vi "Gui4.vi"() -> ()   [LabVIEW 2009]
uses:
  <vilib>/rvi/interface/nirviOpenFPGA/nirviOpenFPGA.xnode
  FPGA Bitfiles/Athena Brain.lvproj_FPGA Target 2_Gray's Mod Motor C~4B.lvbitx
  FPGA/Gray's Mod Motor Controler.vi
  <vilib>/userDefined/High Color/nirio_resource_hc.ctl
  <vilib>/rvi/interface/nirviReadWriteControl/nirviReadWriteControl.xnode
  NiRioSrv.dll
  <vilib>/Utility/error.llb/Error Cluster From Error Code.vi
  <vilib>/rvi/errors/niLvFpgaWhatHappensToTopLevelVI.ctl
  <vilib>/rvi/interface/common/niFpgaNodeNameForErrorReporting.ctl
  <vilib>/rvi/errors/niLvFpgaAdjustHostInterfaceError.vi
  <vilib>/rvi/interface/nirviMethod/nirviMethod.xnode
  <vilib>/rvi/interface/nirviCloseFPGA/nirviCloseFPGA.xnode
  <vilib>/FPGAPlugInAG/sbRIO-9642/nirviIntfOpen_sbRIO-9642.vi
  <vilib>/Utility/error.llb/Merge Errors.vi
  <vilib>/LabVIEW Targets/FPGA/RIO/nirio_HostInterface/nirio_Reset.vi
  <vilib>/LabVIEW Targets/FPGA/RIO/nirio_HostInterface/nirio_DMAStopAll.vi
  <vilib>/LabVIEW Targets/FPGA/RIO/nirio_HostInterface/nirio_DisableInterrupts.vi
  <vilib>/RVI Host/nirviSupport.llb/nirviErrorClusterFromErrorCode.vi
  <vilib>/FPGAPlugInAG/sbRIO-9642/nirviIntfClose_sbRIO-9642.vi
panel:
  out "Restart Loops":bool=TRUE
  in  "Reset Fpga":bool
  in  "stop":bool
  in  "Lidar Enable":bool
  in  "Lidar Output Command":fxp<+/-,20,5> format="%.17g"
  out "Lidar Output Voltage":fxp<+/-,20,5> format="%.17g"
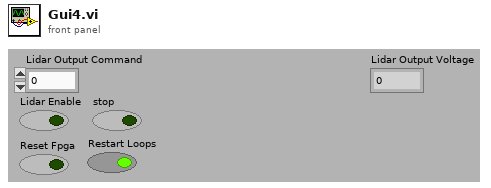
[diagram p1: front panel]
types:
  T1 = typedef "niFpgaNodeNameForErrorReporting.ctl" = enum16{"Open FPGA VI Reference", "Read/Write Control", "Invoke Method: Abort", "Invoke Method: Acknowledge IRQ", "Invoke Method: Download", "Invoke Method: FIFO.Configure", "Invoke Method: FIFO.Read", "Invoke Method: FIFO.Start", "Invoke Method: FIFO.Stop", "Invoke Method: FIFO.Write", "Invoke Method: Reset", "Invoke Method: Run", "Invoke Method: Wait on IRQ", "Close FPGA VI Reference"}
  T2 = typedef "niLvFpgaWhatHappensToTopLevelVI.ctl" = enum16{"top level VI scripted behind XNode", "top level VI inlined behind XNode"}
  T3 = typedef "nirio_resource_hc.ctl" = tag
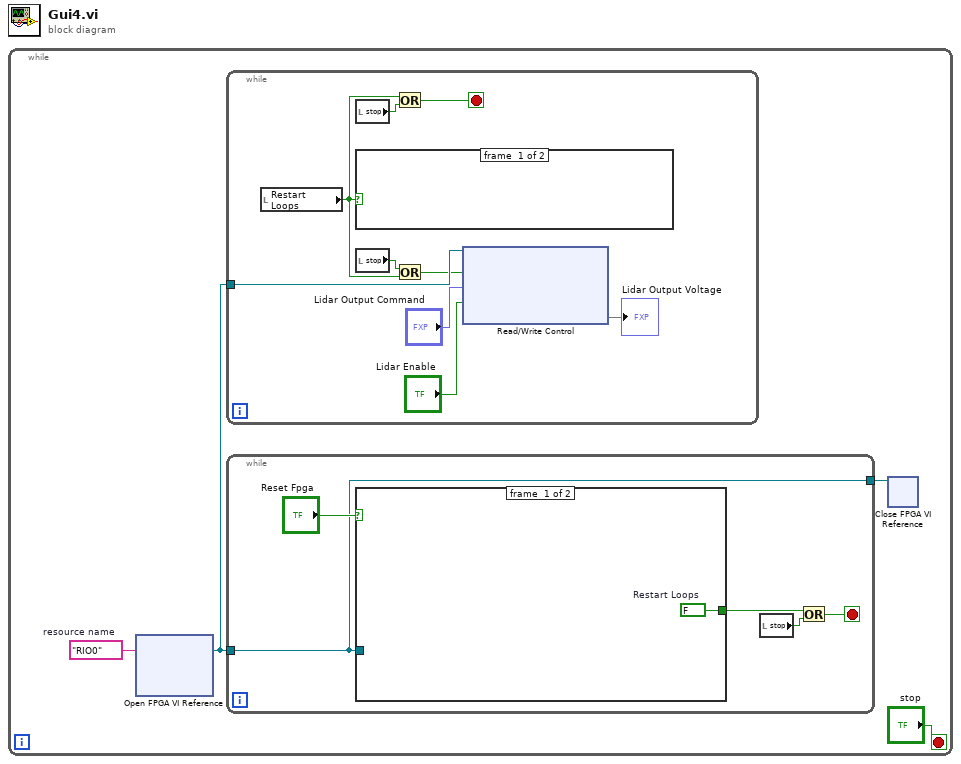
[diagram p0: block diagram]
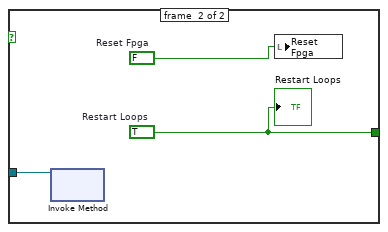
[diagram p2: hidden frame]
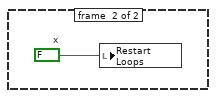
[diagram p3: hidden frame]
diagram:
  n1 = while {
    stop <- "stop" stop-if-true
    w4 = T3 "RIO0"  # resource name
    n2 = xnode "Open FPGA VI Reference"("resource name"=w4) -> ("FPGA VI Reference Out"=w3:refnum<k20>)  [unwired: 1 in, 1 out]
    n3 = while {
      tunnel: w3 -> [w123]
      stop <- w119 stop-if-true
      n4 = local read "Restart Loops"() -> (w120:bool)
      n5 = local read "stop"() -> (w118:bool)
      n6 = case shown="True" w120 {
        frame #0 {
        }
        frame #1 {
          w127 = FALSE  # x
          n7 = local write "Restart Loops"(w127) -> ()
        }
      }
      n8 = local read "stop"() -> (w122:bool)
      n9 = Or(x=w120, y=w118) -> (x .or. y?=w119:bool)
      n10 = Or(x=w122, y=w120) -> (x .or. y?=w121:bool)
      n11 = xnode "Read/Write Control"("FPGA VI Reference In"=w123, "stop"=w121, "Lidar Output Command"="Lidar Output Command", "Lidar Enable"="Lidar Enable") -> ("Lidar Output Voltage"=→"Lidar Output Voltage")  [unwired: 1 in, 2 out]
    }
    n12 = while {
      tunnel: w3 -> [w27]
      tunnel: [w27] -> w2
      stop <- w25 stop-if-true
      n13 = case shown="True" "Reset Fpga" {
        tunnel: w27 -> [_ w32]
        tunnel: [w29 w30] -> w26
        frame #0 {
          w29 = FALSE  # Restart Loops
        }
        frame #1 {
          w30 = TRUE  # Restart Loops
          w31 = FALSE  # Reset Fpga
          n14 = xnode "Invoke Method"("FPGA VI Reference In"=w32) -> ()  [unwired: 1 in, 2 out]
          n15 = local write "Reset Fpga"(w31) -> ()
          "Restart Loops" <- w30
        }
      }
      n16 = local read "stop"() -> (w24:bool)
      n17 = Or(x=w26, y=w24) -> (x .or. y?=w25:bool)
    }
    n18 = xnode "Close FPGA VI Reference"("FPGA VI Reference In"=w2) -> ()  [unwired: 1 in, 1 out]
  }
